vi "Projekt.vi"() -> ()   [LabVIEW 2018]
uses:
  Stany.ctl
panel:
  out "Napiecie ustawione":dbl
  out "Blad multimetr 2":string
  out "Blad multimetr 1":string
  out "Blad zasilacz":string
  out "XY Graph 2":cluster{"X":dbl[], "Y":dbl[]}[](graph) caption="XY Graph"
  out "XY Graph":cluster{"X":dbl[], "Y":dbl[]}[](graph)
  out "I":dbl
  out "V":dbl
  out "Nazwa multimetr 2":string
  out "Nazwa multimetr 1":string
  out "Nazwa zasilacza":string
  in  "VISA resource name 3":refnum<visa-resource-name>
  in  "VISA resource name 2":refnum<visa-resource-name>
  in  "VISA resource name":refnum<visa-resource-name>
  in  "stop":bool
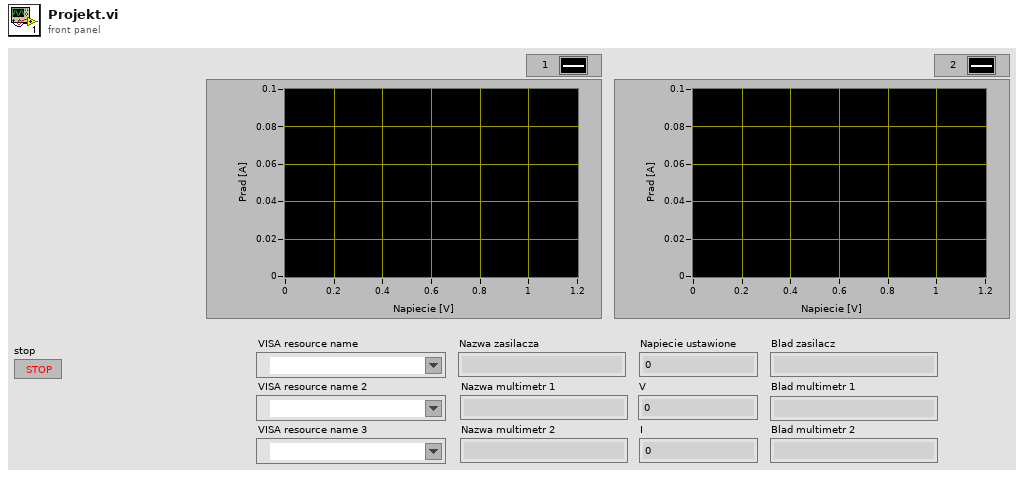
[diagram p1: front panel]
types:
  T1 = enum16{"open", "replace", "create", "open or create", "replace or create", "replace or create with confirmation"}
  T2 = typedef "Stany.ctl" = enum16{"Inicjalizacja", "Ustaw napiecie", "Pomiar I Pomiar U", "Wyswietl na wykresie", "Zapis do pliku", "Koniec", "Zamknij Urzadzenia"}
  T3 = enum16{"Volatage DC", "Current DC", "Resistance"}
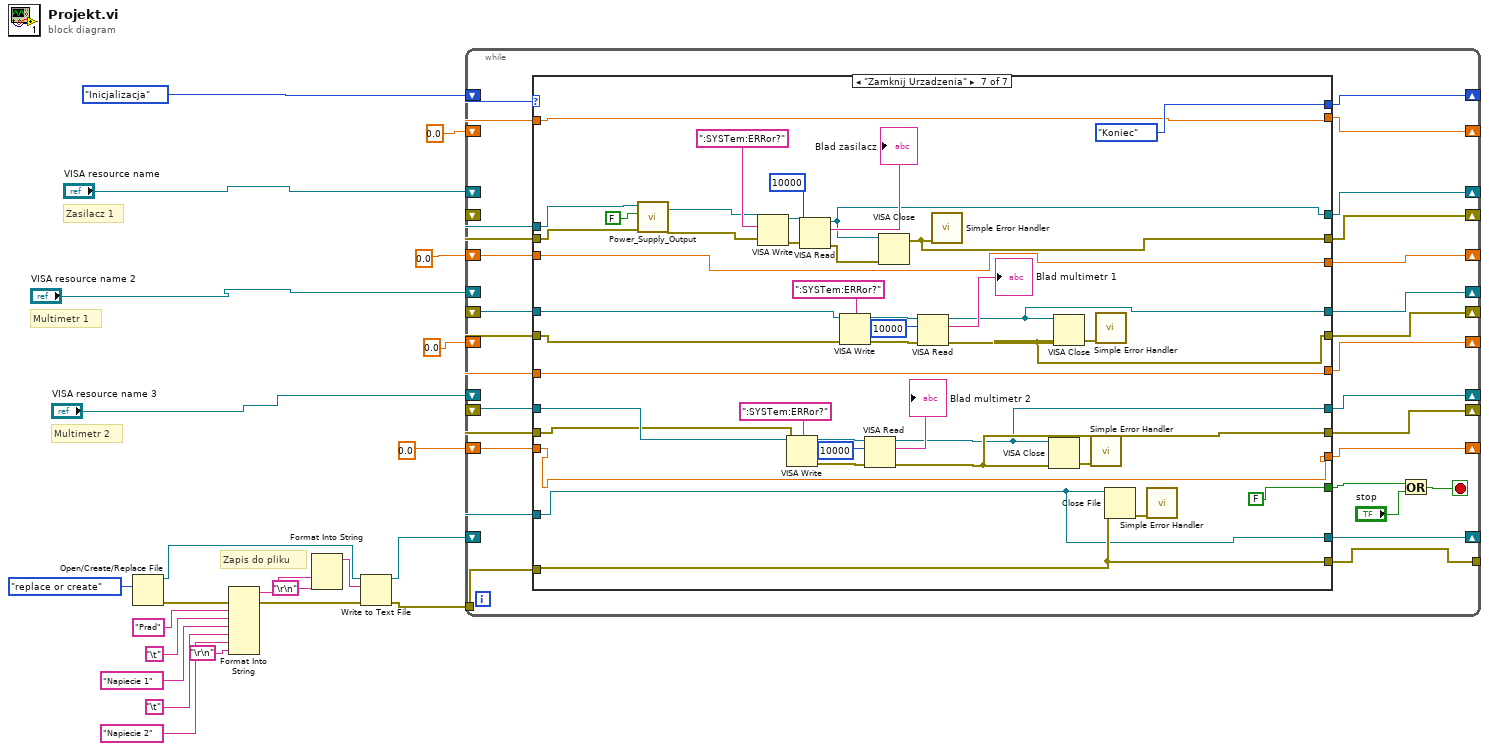
[diagram p0: block diagram]
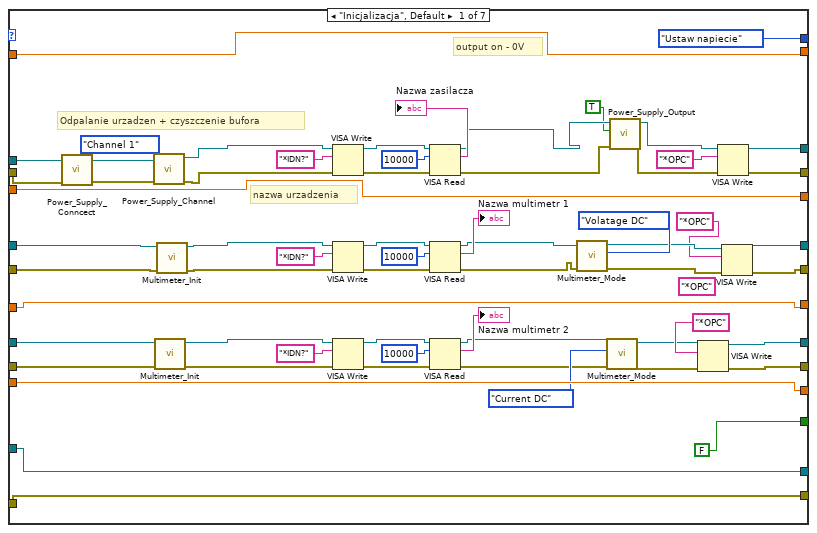
[diagram p2: hidden frame]
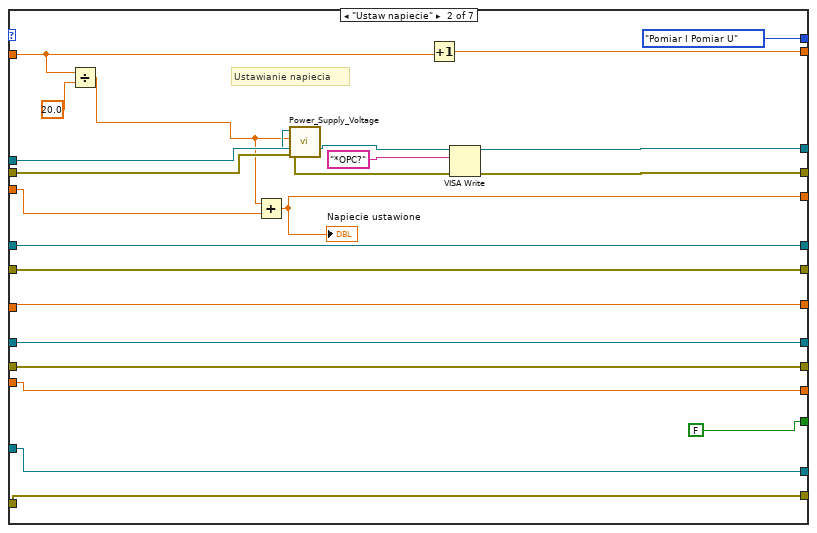
[diagram p3: hidden frame]
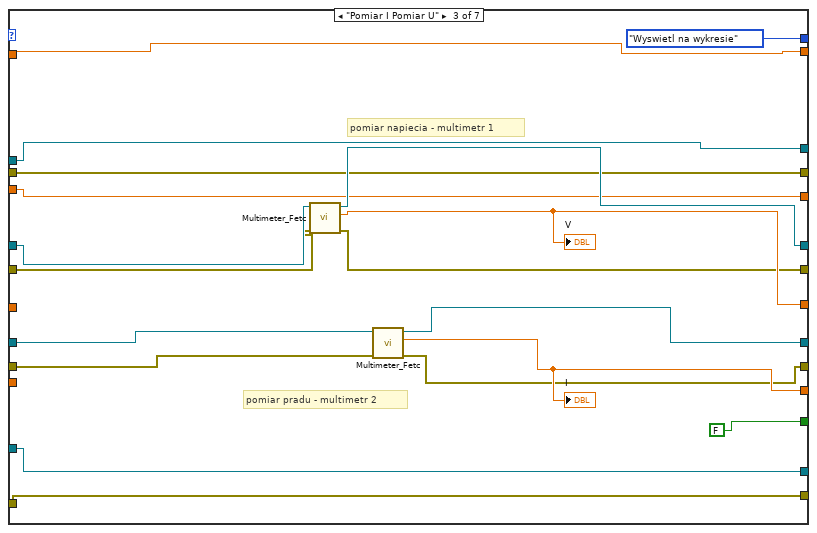
[diagram p4: hidden frame]
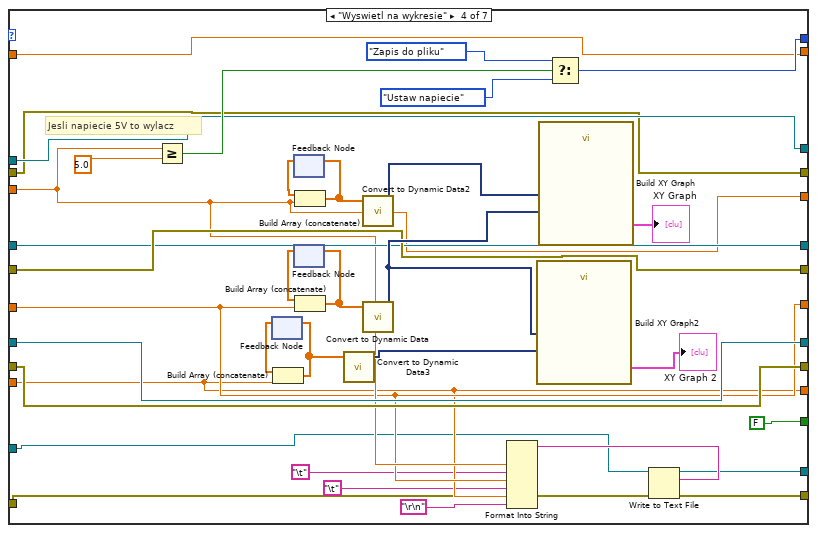
[diagram p5: hidden frame]
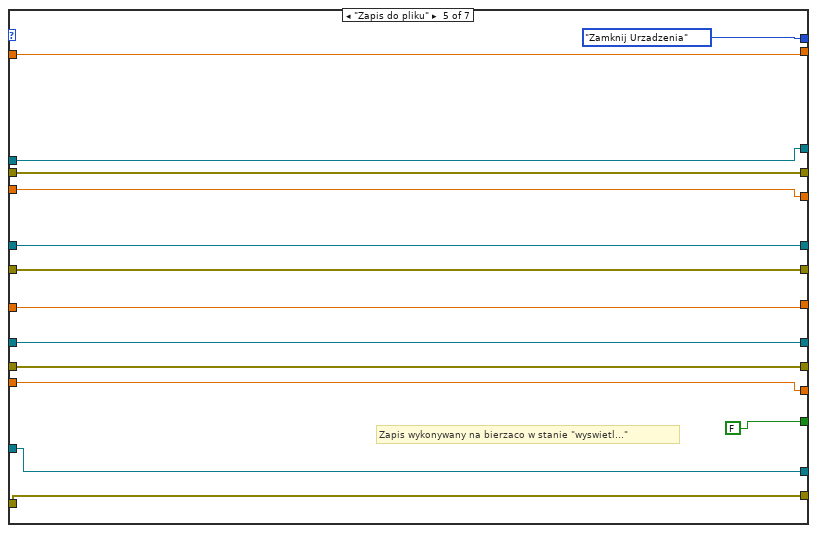
[diagram p6: hidden frame]
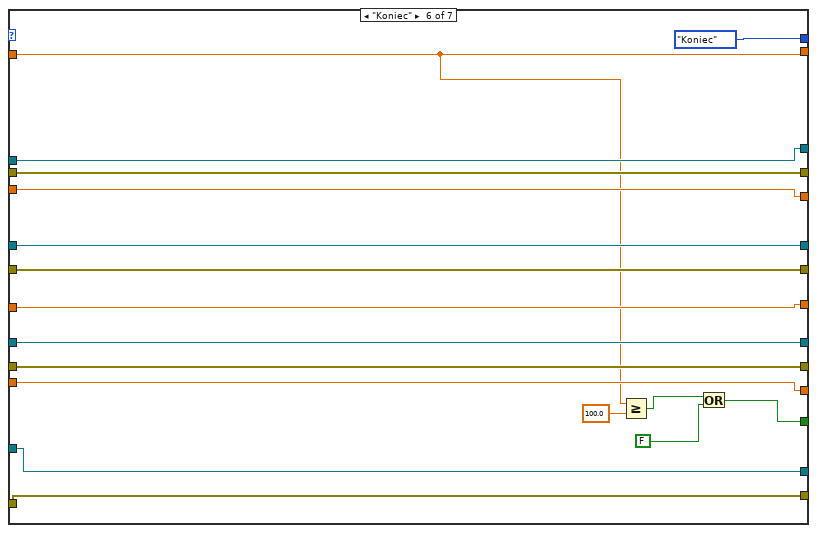
[diagram p7: hidden frame]
diagram:
  # "Zapis do pliku"
  # "Multimetr 2"
  # "Multimetr 1"
  # "Zasilacz 1"
  n1 = Open/Create/Replace File(operation (0:open)=T1."replace or create") -> (refnum out=w17:refnum<file>, error out=w15:errorcluster)  [unwired: 5 in, 1 out]
  n2 = Format Into String(error in=w15, "Prad" ("initial string"), "\t", "Napiecie 1" ("initial string"), "\t", "Napiecie 2" ("initial string"), "\r\n") -> (resulting string=w14:string, error out=w16:errorcluster)  [unwired: 2 in]
  n3 = Format Into String(w14, "\r\n") -> (resulting string=w18:string)  [unwired: 3 in, 1 out]
  n4 = Write to Text File(file (use dialog)=w17, text=w18, error in=w16) -> (refnum out=w4:refnum<file>, error out=w5:errorcluster)  [unwired: 1 in, 1 out]
  n5 = while {
    shift-right: [w51] -> _
    shift-left: Stany."Inicjalizacja" -> [w52]
    shift-right: [w39] -> _
    shift-left: "VISA resource name" -> [w45]
    shift-right: [w41] -> _
    shift-left: "VISA resource name 2" -> [w47]
    shift-right: [w44] -> _
    shift-left: "VISA resource name 3" -> [w49]
    shift-right: [w43] -> _
    shift-left: _ -> [w50]
    shift-right: [w42] -> _
    shift-left: _ -> [w48]
    shift-right: [w40] -> _
    shift-left: _ -> [w46]
    shift-right: [w38] -> _
    shift-left: 0.0 ("y") -> [w37]
    shift-right: [w36] -> _
    shift-left: 0.0 ("y") -> [w33]
    shift-right: [w35] -> _
    shift-left: 0.0 ("y") -> [w32]
    shift-right: [w34] -> _
    shift-left: 0.0 ("y") -> [w31]
    tunnel: w5 -> [w27]
    shift-right: [w26] -> _
    shift-left: w4 -> [w24]
    tunnel: [w25] -> _
    stop <- w30 stop-if-true
    n6 = case shown="\"Zamknij Urzadzenia\"" w52 {
      tunnel: [Stany."Ustaw napiecie" Stany."Pomiar I Pomiar U" Stany."Wyswietl na wykresie" w174 Stany."Zamknij Urzadzenia" Stany."Koniec" Stany."Koniec"] -> w51
      tunnel: [w98 w132 w137 w171 w200 w211 w232] -> w39
      tunnel: [w62 w129 w144 w168 w197 w213 w234] -> w41
      tunnel: [w97 w126 w148 w167 w194 w215 w236] -> w44
      tunnel: w45 -> [w57 w119 w137 w171 w200 w211 w222]
      tunnel: w47 -> [w76 w129 w141 w168 w197 w213 w242]
      tunnel: w49 -> [w82 w126 w146 w167 w194 w215 w240]
      tunnel: w50 -> [w81 w125 w145 w166 w193 w216 w239]
      tunnel: w48 -> [w77 w128 w140 w169 w196 w214 w241]
      tunnel: w46 -> [w80 w120 w138 w170 w199 w212 w221]
      tunnel: [w93 w125 w147 w166 w193 w216 w237] -> w43
      tunnel: [w61 w128 w142 w169 w196 w214 w235] -> w42
      tunnel: [w92 w131 w138 w170 w199 w212 w233] -> w40
      tunnel: w37 -> [w90 w117 w152 w172 w201 w207 w229]
      tunnel: [w90 w135 w152 w172 w201 w207 w229] -> w38
      tunnel: [w89 w114 w139 w165 w198 w219 w231] -> w36
      tunnel: [w88 w127 w143 w164 w195 w218 w230] -> w35
      tunnel: [w87 w124 w149 w163 w192 w217 w238] -> w34
      tunnel: w33 -> [w89 w115 w139 w165 w198 w219 w231]
      tunnel: w32 -> [w88 w127 _ w164 w195 w218 w230]
      tunnel: w31 -> [w87 w124 _ w163 w192 w217 w238]
      tunnel: [FALSE FALSE FALSE FALSE FALSE w206 FALSE] -> w28
      tunnel: w27 -> [w85 w122 w150 w158 w190 w209 w227]
      tunnel: [w86 w123 w151 w157 w191 w210 w226] -> w26
      tunnel: [w85 w122 w150 w156 w190 w209 w227] -> w25
      tunnel: w24 -> [w86 w123 w151 w155 w191 w210 w226]
      frame "Inicjalizacja", Default {
        (unwired) "*OPC" ("write buffer")
        # "output on - 0V"
        # "nazwa urzadzenia"
        # "Odpalanie urzadzen + czyszczenie bufora"
        n7 = call "Power_Supply_Conncect.vi"("error in"=w80) -> ("error out"=w54:errorcluster)  [unwired: 9 in, 1 out]
        n8 = call "Power_Supply_Channel.vi"("error in"=w54, "Channel"=enum16{"Channel 1", "Channel 2"}."Channel 1", "VISA resource name"=w57) -> ("error out"=w55:errorcluster, "VISA resource name out"=w56:refnum<visa-resource-name>)  [unwired: 7 in]
        n9 = call "Multimeter_Init.vi"("error in"=w81, "VISA resource name"=w82) -> ("error out"=w83:errorcluster, "VISA resource name out"=w84:refnum<visa-resource-name>)  [unwired: 8 in]
        n10 = call "Multimeter_Init.vi"("error in"=w77, "VISA resource name"=w76) -> ("error out"=w78:errorcluster, "VISA resource name out"=w79:refnum<visa-resource-name>)  [unwired: 8 in]
        n11 = VISA Write(VISA resource name=w56, write buffer="*IDN?", error in (no error)=w55) -> (VISA resource name out=w108:refnum<visa-resource-name>, error out=w94:errorcluster)  [unwired: 1 out]
        n12 = VISA Write(VISA resource name=w79, write buffer="*IDN?", error in (no error)=w78) -> (VISA resource name out=w106:refnum<visa-resource-name>, error out=w95:errorcluster)  [unwired: 1 out]
        n13 = VISA Write(VISA resource name=w84, write buffer="*IDN?", error in (no error)=w83) -> (VISA resource name out=w104:refnum<visa-resource-name>, error out=w96:errorcluster)  [unwired: 1 out]
        n14 = VISA Read(VISA resource name=w108, byte count=u32 10000, error in (no error)=w94) -> (VISA resource name out=w75:refnum<visa-resource-name>, read buffer=→"Nazwa zasilacza":string, error out=w74:errorcluster)  [unwired: 1 out]
        n15 = VISA Read(VISA resource name=w106, byte count=u32 10000, error in (no error)=w95) -> (VISA resource name out=w69:refnum<visa-resource-name>, read buffer=→"Nazwa multimetr 1":string, error out=w68:errorcluster)  [unwired: 1 out]
        n16 = VISA Read(VISA resource name=w104, byte count=u32 10000, error in (no error)=w96) -> (VISA resource name out=w64:refnum<visa-resource-name>, read buffer=→"Nazwa multimetr 2":string, error out=w65:errorcluster)  [unwired: 1 out]
        n17 = call "Multimeter_Mode.vi"("error in"=w68, "Multimeter function select"=T3."Volatage DC", "VISA resource name"=w69) -> ("error out"=w59:errorcluster, "VISA resource name out"=w60:refnum<visa-resource-name>)  [unwired: 7 in]
        n18 = call "Multimeter_Mode.vi"("error in"=w65, "Multimeter function select"=T3."Current DC", "VISA resource name"=w64) -> ("error out"=w66:errorcluster, "VISA resource name out"=w63:refnum<visa-resource-name>)  [unwired: 7 in]
        n19 = call "Power_Supply_Output.vi"("error in (no error)"=w74, "Output"=TRUE, "VISA resource name"=w75) -> ("error out"=w72:errorcluster, "VISA resource name out"=w73:refnum<visa-resource-name>)  [unwired: 7 in]
        n20 = VISA Write(VISA resource name=w63, write buffer="*OPC", error in (no error)=w66) -> (VISA resource name out=w97:refnum<visa-resource-name>, error out=w93:errorcluster)  [unwired: 1 out]
        n21 = VISA Write(VISA resource name=w73, write buffer="*OPC", error in (no error)=w72) -> (VISA resource name out=w98:refnum<visa-resource-name>, error out=w92:errorcluster)  [unwired: 1 out]
        n22 = VISA Write(VISA resource name=w60, write buffer="*OPC", error in (no error)=w59) -> (VISA resource name out=w62:refnum<visa-resource-name>, error out=w61:errorcluster)  [unwired: 1 out]
      }
      frame "Ustaw napiecie" {
        # "Ustawianie napiecia"
        n23 = Divide(x=w117, y=20.0) -> (x/y=w116:dbl)
        n24 = Add(x=w116, y=w115) -> (x+y=w114:dbl)
        "Napiecie ustawione" <- w114
        n25 = call "Power_Supply_Voltage.vi"("error in (no error)"=w120, "Voltage"=w116, "VISA resource name"=w119) -> ("error out"=w121:errorcluster, "VISA resource name out"=w118:refnum<visa-resource-name>)  [unwired: 7 in]
        n26 = Increment(x=w117) -> (x+1=w135:dbl)
        n27 = VISA Write(VISA resource name=w118, write buffer="*OPC?", error in (no error)=w121) -> (VISA resource name out=w132:refnum<visa-resource-name>, error out=w131:errorcluster)  [unwired: 1 out]
      }
      frame "Pomiar I Pomiar U" {
        # "pomiar pradu - multimetr 2"
        # "pomiar napiecia - multimetr 1"
        n28 = call "Multimeter_Fetc.vi"("error in"=w140, "VISA resource name"=w141) -> ("error out"=w142:errorcluster, "Measurement result"=w143:dbl, "VISA resource name out"=w144:refnum<visa-resource-name>)  [unwired: 7 in]
        "V" <- w143
        n29 = call "Multimeter_Fetc.vi"("error in"=w145, "VISA resource name"=w146) -> ("error out"=w147:errorcluster, "Measurement result"=w149:dbl, "VISA resource name out"=w148:refnum<visa-resource-name>)  [unwired: 7 in]
        "I" <- w149
      }
      frame "Wyswietl na wykresie" {
        # "Jesli napiecie 5V to wylacz"
        n30 = Greater Or Equal?(x=w165, y=5.0 ("x")) -> (x >= y?=w178:bool)
        n31 = feedback #1() -> (w183:dbl[])  [unwired: 1 in]
        n32 = Build Array (concatenate)(w183, w163) -> (w182:dbl[])
        n33 = feedback-in #1(w182) -> ()
        n34 = feedback #2() -> (w185:dbl[])  [unwired: 1 in]
        n35 = feedback #3() -> (w184:dbl[])  [unwired: 1 in]
        n36 = Build Array (concatenate)(w185, w165) -> (w189:dbl[])
        n37 = feedback-in #2(w189) -> ()
        n38 = Build Array (concatenate)(w184, w164) -> (w188:dbl[])
        n39 = feedback-in #3(w188) -> ()
        n40 = call "Convert to Dynamic Data3"("Array"=w182) -> ("Dynamic Data Type"=w180:dynamicdata)  [unwired: 3 in]
        n41 = call "Convert to Dynamic Data2"("Array"=w189) -> ("Dynamic Data Type"=w187:dynamicdata)  [unwired: 3 in]
        n42 = call "Convert to Dynamic Data"("Array"=w188) -> ("Dynamic Data Type"=w181:dynamicdata)  [unwired: 3 in]
        n43 = Format Into String(w165, "\t", w164, "\t", w163, "\r\n") -> (resulting string=w159:string)  [unwired: 3 in, 1 out]
        n44 = call "Build XY Graph2"("Y Input"=w180, "X Input"=w181) -> ("XY Graph"=→"XY Graph 2":cluster{"X":dbl[], "Y":dbl[]}[])  [unwired: 8 in, 1 out]
        n45 = call "Build XY Graph"("Y Input"=w181, "X Input"=w187) -> ("XY Graph"=→"XY Graph":cluster{"X":dbl[], "Y":dbl[]}[])  [unwired: 8 in, 1 out]
        n46 = Select(t=Stany."Zapis do pliku", s=w178, f=Stany."Ustaw napiecie") -> (s? t:f=w174:T2)
        n47 = Write to Text File(file (use dialog)=w155, text=w159, error in=w158) -> (refnum out=w157:refnum<file>, error out=w156:errorcluster)  [unwired: 1 in, 1 out]
      }
      frame "Zapis do pliku" {
        # "Zapis wykonywany na bierzaco w stanie \"wyswietl...\""
      }
      frame "Koniec" {
        n48 = Greater Or Equal?(x=w207, y=100.0) -> (x >= y?=w205:bool)
        n49 = Or(x=w205, y=FALSE) -> (x .or. y?=w206:bool)
      }
      frame "Zamknij Urzadzenia" {
        n50 = call "Power_Supply_Output.vi"("error in (no error)"=w221, "Output"=FALSE, "VISA resource name"=w222) -> ("error out"=w223:errorcluster, "VISA resource name out"=w224:refnum<visa-resource-name>)  [unwired: 7 in]
        n51 = VISA Write(VISA resource name=w224, write buffer=":SYSTem:ERRor?", error in (no error)=w223) -> (VISA resource name out=w259:refnum<visa-resource-name>, error out=w258:errorcluster)  [unwired: 1 out]
        n52 = VISA Write(VISA resource name=w240, write buffer=":SYSTem:ERRor?", error in (no error)=w239) -> (VISA resource name out=w247:refnum<visa-resource-name>, error out=w248:errorcluster)  [unwired: 1 out]
        n53 = VISA Read(VISA resource name=w259, byte count=u32 10000, error in (no error)=w258) -> (VISA resource name out=w232:refnum<visa-resource-name>, read buffer=→"Blad zasilacz":string, error out=w257:errorcluster)  [unwired: 1 out]
        n54 = VISA Write(VISA resource name=w242, write buffer=":SYSTem:ERRor?", error in (no error)=w241) -> (VISA resource name out=w254:refnum<visa-resource-name>, error out=w253:errorcluster)  [unwired: 1 out]
        n55 = VISA Read(VISA resource name=w247, byte count=u32 10000, error in (no error)=w248) -> (VISA resource name out=w236:refnum<visa-resource-name>, read buffer=→"Blad multimetr 2":string, error out=w237:errorcluster)  [unwired: 1 out]
        n56 = VISA Close(VISA resource name=w232, error in (no error)=w257) -> (error out=w233:errorcluster)
        n57 = VISA Read(VISA resource name=w254, byte count=u32 10000, error in (no error)=w253) -> (VISA resource name out=w234:refnum<visa-resource-name>, read buffer=→"Blad multimetr 1":string, error out=w235:errorcluster)  [unwired: 1 out]
        n58 = call <vilib>:"Simple Error Handler.vi"("error in (no error)"=w233) -> ()  [unwired: 4 in, 5 out]
        n59 = VISA Close(VISA resource name=w236, error in (no error)=w237) -> (error out=w245:errorcluster)
        n60 = VISA Close(VISA resource name=w234, error in (no error)=w235) -> (error out=w262:errorcluster)
        n61 = call <vilib>:"Simple Error Handler.vi"("error in (no error)"=w245) -> ()  [unwired: 4 in, 5 out]
        n62 = call <vilib>:"Simple Error Handler.vi"("error in (no error)"=w262) -> ()  [unwired: 4 in, 5 out]
        n63 = Close File(refnum=w226, error in=w227) -> (error out=w228:errorcluster)  [unwired: 1 out]
        n64 = call <vilib>:"Simple Error Handler.vi"("error in (no error)"=w228) -> ()  [unwired: 4 in, 5 out]
      }
    }
    n65 = Or(x=w28, y="stop") -> (x .or. y?=w30:bool)
  }
